vi "Cnvrt X SI units.vi"(0 "reference in":refnum<class "XYgraph.lvclass">, 2 "X Units (micro)":T1="micro", 5 "error in (no error)":errorcluster) -> (14 "reference out":refnum<class "XYgraph.lvclass">, 19 "error out":errorcluster)   [LabVIEW 2019, in "XYgraph.lvclass"]
doc: "Changes the SI units of an X axis"
uses:
  XYgraph.lvclass
  Units --enum.ctl
  <vilib>/Utility/miscctls.llb/LVOffsetAndMultiplierTypeDef.ctl
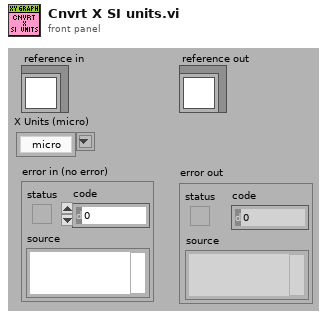
[diagram p1: front panel]
types:
  T1 = typedef "XYgraph.lvclass/Units --enum.ctl" = string
  T2 = typedef "LVOffsetAndMultiplierTypeDef.ctl" = cluster{"Offset":dbl, "Multiplier":dbl}
  T3 = typedef "XYgraph.lvclass/ObjectAttributes.ctl" = cluster{"FPref":T4, "MyAttribute":dbl, "X multiplier":dbl, "Y multiplier":dbl, "X Scale name":string, "Y Scale name":string, "Fcurve metadata":T5, "Fcurve":refnum<class "Fcurve.lvclass">}
  T4 = typedef "XYgraph.lvclass/XY graph ref.ctl" = refnum<vi>
  T5 = typedef "Fcurve.lvclass/Metadata.ctl" = cluster{"dt (us)":dbl, "Dec Factor":dbl, "Z piezo Sensitivity (nm/V)":dbl, "K (N/m)":dbl, "Sp (V)":dbl, "Contact (ms)":dbl, "Zpos contact":dbl, "Vel_app (nm/s)":dbl, "Vel_ret (nm/s)":dbl, "deltaV (nm)":dbl, "Def_V0 (v)":dbl, "Piezo gain":dbl, "invOLS (nm/V)":dbl}
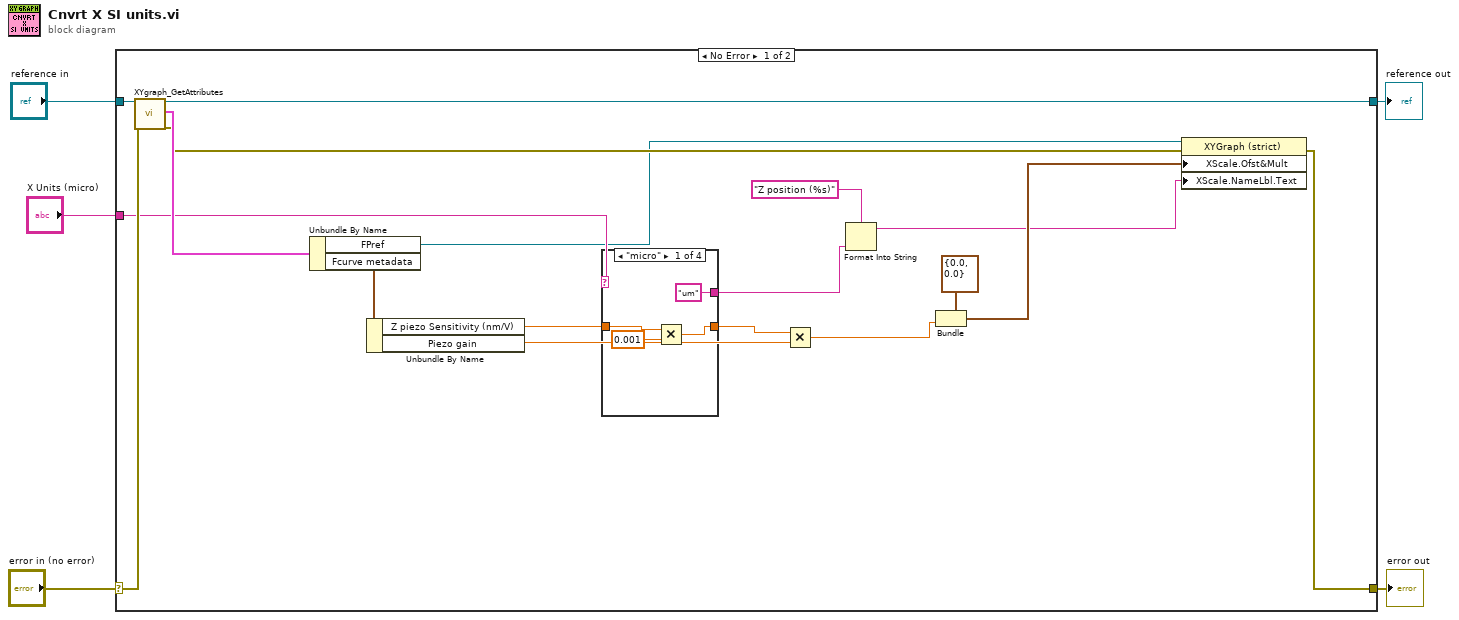
[diagram p0: block diagram]
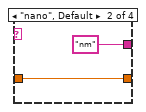
[diagram p2: hidden frame]
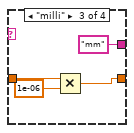
[diagram p3: hidden frame]
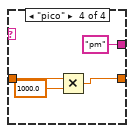
[diagram p4: hidden frame]
diagram:
  n1 = case shown="No Error" "error in (no error)" {
    selector: "error in (no error)" -> [w23 w39]
    tunnel: [w13 w39] -> w4
    tunnel: [w8 w38] -> w2
    tunnel: "reference in" -> [w22 w38]
    tunnel: "X Units (micro)" -> [w16 _]
    frame No Error {
      n2 = call "XYgraph_GetAttributes.vi"("reference in"=w22, "error in (no error)"=w23) -> ("reference out"=w8:refnum<class "XYgraph.lvclass">, "attributes"=w17:T3, "error out"=w7:errorcluster)  [unwired: 14 in, 1 out]
      n3 = Unbundle By Name(w17) -> ("FPref"=w6:T4, "Fcurve metadata"=w9:T5)
      n4 = Unbundle By Name(w9) -> ("Z piezo Sensitivity (nm/V)"=w15:dbl, "Piezo gain"=w21:dbl)
      n5 = case shown="\"micro\"" w16 {
        tunnel: w15 -> [w27 w29 w33 w37]
        tunnel: [w26 w29 w32 w36] -> w14
        tunnel: ["um" ("input 1") "nm" ("input 1") "mm" ("input 1") "pm" ("input 1")] -> w10
        frame "micro" {
          n6 = Multiply(x=w27, y=0.001) -> (x*y=w26:dbl)
        }
        frame "nano", Default {
        }
        frame "milli" {
          n7 = Multiply(x=w33, y=1e-06) -> (x*y=w32:dbl)
        }
        frame "pico" {
          n8 = Multiply(x=w37, y=1000.0) -> (x*y=w36:dbl)
        }
      }
      n9 = Multiply(x=w14, y=w21) -> (x*y=w18:dbl)
      n10 = Format Into String(format string="Z position (%s)" ("X Scale.Name Label.Text"), w10) -> (resulting string=w11:string)  [unwired: 2 in, 1 out]
      n11 = Bundle(cluster=T2 {"Offset"=0.0, "Multiplier"=0.0} ("X Scale.Offset and Multiplier"), "Multiplier"=w18) -> (w20:T2)  [unwired: 1 in]
      n12 = property on="Property Node" class="XYGraph (strict)"(reference=w6, error in=w7, "XScale.Ofst&Mult"=w20, "XScale.NameLbl.Text"=w11) -> (error out=w13:errorcluster)  [unwired: 1 out]
    }
    frame Error {
    }
  }
  "error out" <- w4
  "reference out" <- w2
